vi "Report_Array_Spliting.vi"(8 "Input array 2":string[][](array[string]), 9 "columns Header":string[](array[string]), 10 "Machine Selection":string(combo)="ALL STATION") -> (1 "collumns Header out":string[](array[string]), 2 "Output":string[][](array[string]))   [LabVIEW 2017]
uses:
  <userlib>/_OpenG.lib/array/array.llb/Search 1D Array (String)__ogtk.vi
  <userlib>/_OpenG.lib/array/array.llb/Delete Elements from 2D Array (String)__ogtk.vi
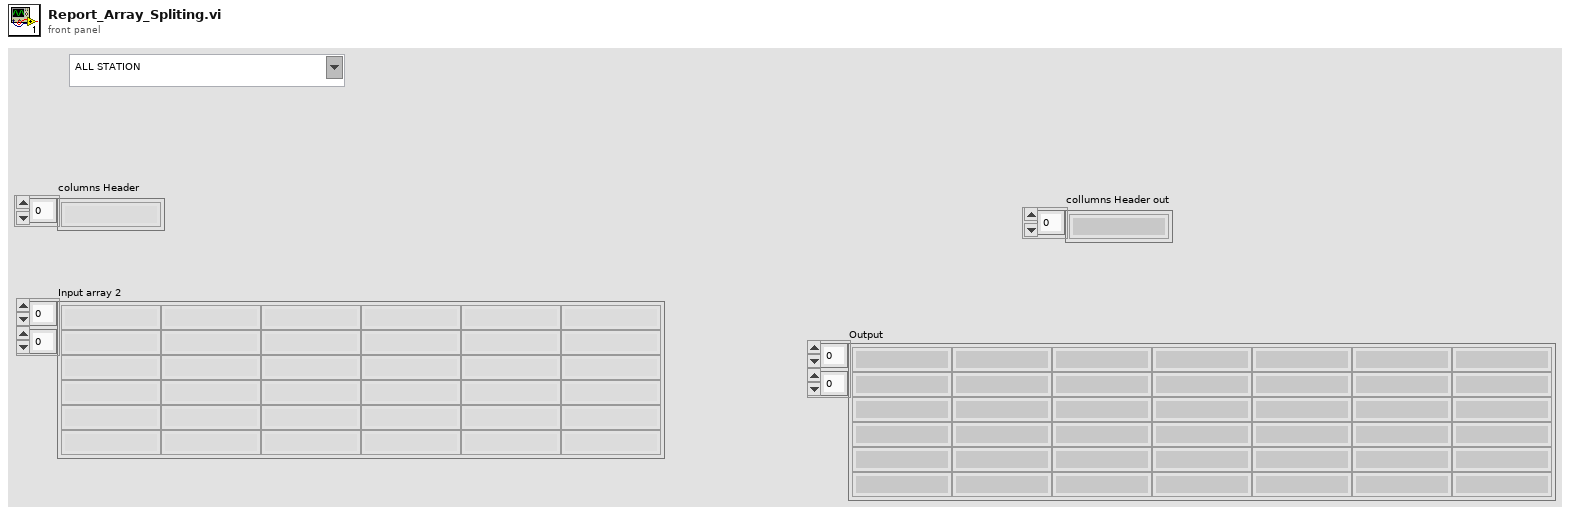
[diagram p1: front panel]
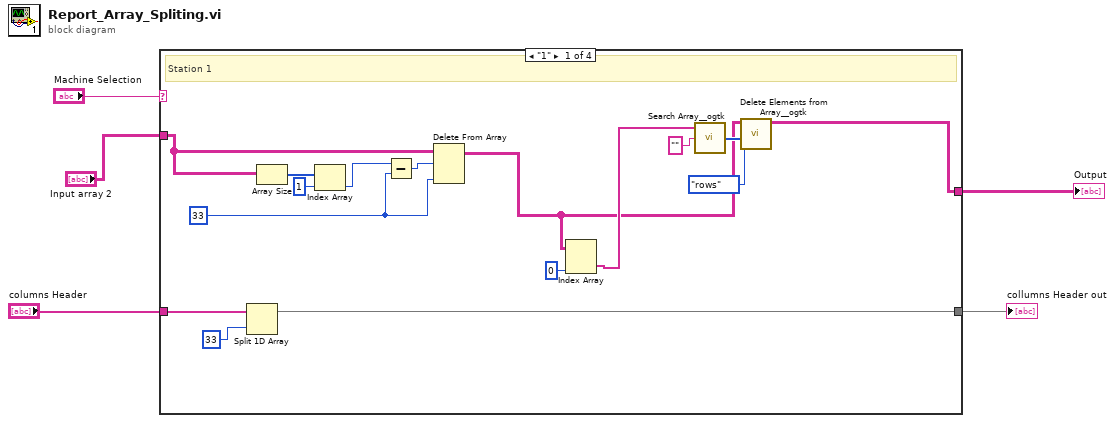
[diagram p0: block diagram]
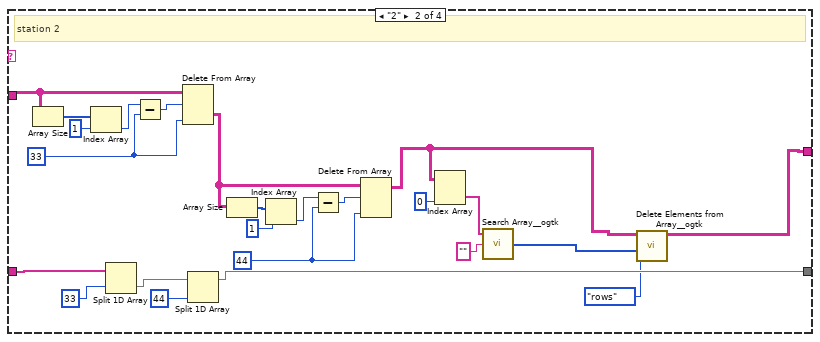
[diagram p2: hidden frame]
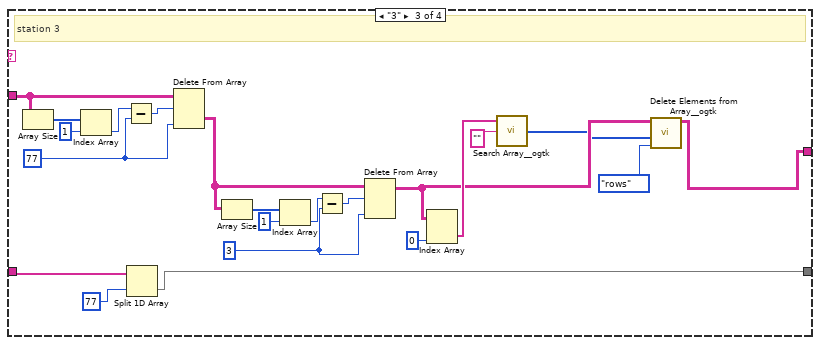
[diagram p3: hidden frame]
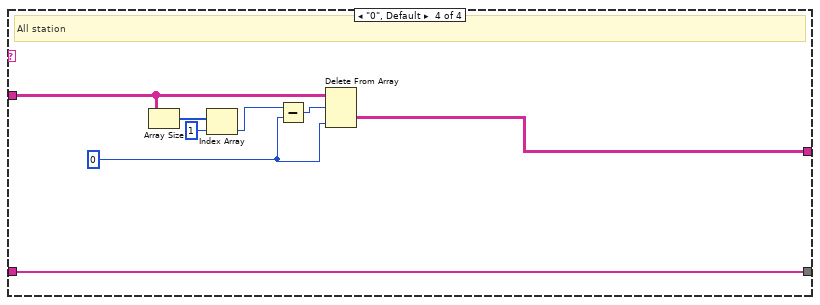
[diagram p4: hidden frame]
diagram:
  n1 = case shown="\"1\"" "Machine Selection" {
    tunnel: "Input array 2" -> [w16 w40 w57 w70]
    tunnel: [w8 w22 w48 w69] -> w3
    tunnel: "columns Header" -> [w15 w32 w54 w68]
    tunnel: [w13 w29 w53 w68] -> w1
    frame "1" {
      w17 = 33 ("index COLUMN 2")
      # "Station 1"
      n2 = Split 1D Array(array=w15, index=33 ("index COLUMN 2")) -> (first subarray=w13:string[])  [unwired: 1 out]
      n3 = Array Size(array=w16) -> (size(s)=w21:i32[])
      n4 = Index Array(array=w21, index=1) -> (element=w19:i32)
      n5 = Subtract(x=w19, y=w17) -> (x-y=w20:i32)
      n6 = Delete From Array(array=w16, length=w20, index (col)=w17) -> (array with subset deleted=w6:string[][])  [unwired: 1 in, 1 out]
      n7 = Index Array(array=w6, index (col)=0 ("index (row)")) -> (element=w7:string[])  [unwired: 1 in]
      n8 = call-poly <userlib>:"Search Array__ogtk.vi"("Array"=w7, "Element Data"="" ("element")) -> ("Indices of Elements"=w11:i32[])  [unwired: 7 in]
      n9 = call-poly <userlib>:"Delete Elements from Array__ogtk.vi"("delete (rows or columns)"=enum16{"rows", "columns"}."rows", "indices"=w11, "array"=w6) -> ("array w/ subset deleted"=w8:string[][])  [unwired: 7 in, 1 out]
    }
    frame "2" {
      w35 = 44 ("index COLUMN 2")
      w41 = 33 ("index COLUMN 2")
      # "station 2"
      n10 = Array Size(array=w40) -> (size(s)=w45:i32[])
      n11 = Index Array(array=w45, index=1) -> (element=w43:i32)
      n12 = Split 1D Array(array=w32, index=33 ("index COLUMN 2")) -> (second subarray=w30:string[])  [unwired: 1 out]
      n13 = Subtract(x=w43, y=w41) -> (x-y=w44:i32)
      n14 = Delete From Array(array=w40, length=w44, index (col)=w41) -> (deleted portion=w34:string[][])  [unwired: 1 in, 1 out]
      n15 = Split 1D Array(array=w30, index=44 ("index COLUMN 2")) -> (first subarray=w29:string[])  [unwired: 1 out]
      n16 = Array Size(array=w34) -> (size(s)=w36:i32[])
      n17 = Index Array(array=w36, index=1) -> (element=w38:i32)
      n18 = Subtract(x=w38, y=w35) -> (x-y=w37:i32)
      n19 = Delete From Array(array=w34, length=w37, index (col)=w35) -> (array with subset deleted=w23:string[][])  [unwired: 1 in, 1 out]
      n20 = Index Array(array=w23, index (col)=0 ("index (row)")) -> (element=w24:string[])  [unwired: 1 in]
      n21 = call-poly <userlib>:"Search Array__ogtk.vi"("Array"=w24, "Element Data"="" ("element")) -> ("Indices of Elements"=w27:i32[])  [unwired: 7 in]
      n22 = call-poly <userlib>:"Delete Elements from Array__ogtk.vi"("delete (rows or columns)"=enum16{"rows", "columns"}."rows", "indices"=w27, "array"=w23) -> ("array w/ subset deleted"=w22:string[][])  [unwired: 7 in, 1 out]
    }
    frame "3" {
      w60 = 3 ("index COLUMN 2")
      w58 = 77 ("index COLUMN 2")
      # "station 3"
      n23 = Array Size(array=w57) -> (size(s)=w67:i32[])
      n24 = Index Array(array=w67, index=1) -> (element=w65:i32)
      n25 = Subtract(x=w65, y=w58) -> (x-y=w66:i32)
      n26 = Split 1D Array(array=w54, index=77 ("index COLUMN 2")) -> (second subarray=w53:string[])  [unwired: 1 out]
      n27 = Delete From Array(array=w57, length=w66, index (col)=w58) -> (deleted portion=w56:string[][])  [unwired: 1 in, 1 out]
      n28 = Array Size(array=w56) -> (size(s)=w62:i32[])
      n29 = Index Array(array=w62, index=1) -> (element=w64:i32)
      n30 = Subtract(x=w64, y=w60) -> (x-y=w63:i32)
      n31 = Delete From Array(array=w56, length=w63, index (col)=w60) -> (array with subset deleted=w49:string[][])  [unwired: 1 in, 1 out]
      n32 = Index Array(array=w49, index (col)=0 ("index (row)")) -> (element=w51:string[])  [unwired: 1 in]
      n33 = call-poly <userlib>:"Search Array__ogtk.vi"("Array"=w51, "Element Data"="" ("element")) -> ("Indices of Elements"=w46:i32[])  [unwired: 7 in]
      n34 = call-poly <userlib>:"Delete Elements from Array__ogtk.vi"("delete (rows or columns)"=enum16{"rows", "columns"}."rows", "indices"=w46, "array"=w49) -> ("array w/ subset deleted"=w48:string[][])  [unwired: 7 in, 1 out]
    }
    frame "0", Default {
      w71 = 0 ("index COLUMN 2")
      # "All station"
      n35 = Array Size(array=w70) -> (size(s)=w75:i32[])
      n36 = Index Array(array=w75, index=1) -> (element=w73:i32)
      n37 = Subtract(x=w73, y=w71) -> (x-y=w74:i32)
      n38 = Delete From Array(array=w70, length=w74, index (col)=w71) -> (deleted portion=w69:string[][])  [unwired: 1 in, 1 out]
    }
  }
  "Output" <- w3
  "collumns Header out" <- w1
